vi "I2COUSBProxy.vi"(8 "error in (no error)":errorcluster, 11 "I2COOUSBParams":T1) -> (0 "error out":errorcluster, 3 "CameraTestingProxy":refnum<class "CameraTestingProxyAPI.lvclass">)   [LabVIEW 2020, in "CamTestProxyLdr.lvlib"]
uses:
  CamTestProxyLdr.lvlib
  bin/CameraTestingProxy/CameraTestingProxy.lvlibp/CameraTestingProxyAPI/CameraTestingProxyAPI.lvclass
  bin/Camera/ICamera.lvlibp/ICamera/ICamera.lvclass
  bin/CameraTestingApp/ICameraTesting_typedef.lvlibp/CameraInfo.ctl
  bin/CameraTestingApp/ICameraTesting_typedef.lvlibp
  bin/Camera/CameraI2COUSB.lvlibp/Camera/CameraI2COUSB.lvclass
  bin/CameraTestingApp/CameraTesting.lvlibp/CameraTesting/CameraTesting.lvclass
  E:/GitHub/Evaluation_Test/Teststand/Code_Modules/bin/Camera/CameraI2COUSB.lvlibp/Camera/CameraI2COUSB.lvclass
  E:/GitHub/Evaluation_Test/Teststand/Code_Modules/bin/Camera/ICamera.lvlibp/ICamera/ICamera.lvclass
  E:/GitHub/Evaluation_Test/Teststand/Code_Modules/bin/Actor Framework/Actor Framework.lvlibp/1abvi3w/vi.lib/ActorFramework/Actor/Actor.lvclass
  E:/GitHub/Evaluation_Test/Teststand/Code_Modules/bin/CameraTestingApp/CameraTesting.lvlibp/CameraTesting/CameraTesting.lvclass
  E:/GitHub/Evaluation_Test/Teststand/Code_Modules/bin/CameraTestingApp/ICameraTesting.lvlibp/ICameraTesting/ICameraTesting.lvclass
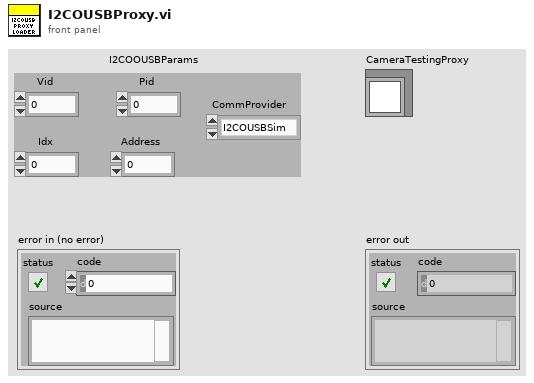
[diagram p1: front panel]
types:
  T1 = cluster{"Vid":u32, "Pid":u32, "Idx":u32, "Address":u32, "CommProvider":enum16{"I2COUSBSim", "ProdType_1", "ProdType_2", "Prod_Type_i", "ProdType_n"}}
  T2 = typedef "ICameraTesting_typedef.lvlibp/CameraInfo.ctl" = cluster{"ICamera ":refnum<class "ICamera.lvclass">, "Connection String":string}
  T3 = enum16{"I2COUSBSim", "ProdType_1", "ProdType_2", "Prod_Type_i", "ProdType_n"}
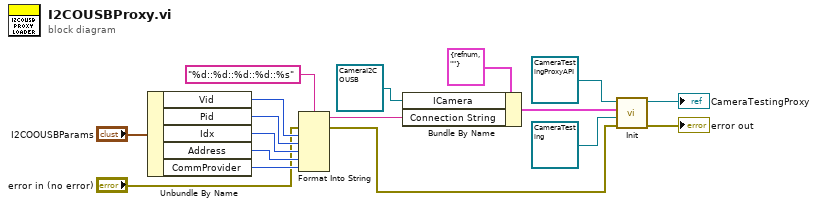
[diagram p0: block diagram]
diagram:
  n1 = Unbundle By Name("I2COOUSBParams") -> ("Vid"=w16:u32, "Pid"=w15:u32, "Idx"=w14:u32, "Address"=w13:u32, "CommProvider"=w12:T3)
  n2 = Format Into String(format string="%d::%d::%d::%d::%s", error in="error in (no error)", w16, w15, w14, w13, w12) -> (resulting string=w9:string, error out=w4:errorcluster)  [unwired: 1 in]
  n3 = Bundle By Name(cluster=T2 {"ICamera "=refnum, "Connection String"=""} ("CameraInfo"), "ICamera"=refnum<class "CameraI2COUSB.lvclass"> refnum ("CameraI2COUSB.lvlibp:CameraI2COUSB.lvclass"), "Connection String"=w9) -> (w6:T2)
  n4 = call-dynamic "Init.vi"("error in (no error)"=w4, "ICameraTesting"=refnum<class "CameraTesting.lvclass"> refnum ("CameraTesting.lvlibp:CameraTesting.lvclass"), "CameraInfo"=w6, "CameraTestingProxy"=refnum<class "CameraTestingProxyAPI.lvclass"> refnum) -> ("error out"=→"error out":errorcluster, "CameraTestingProxy"=→"CameraTestingProxy":refnum<class "CameraTestingProxyAPI.lvclass">)  [unwired: 6 in]
